vi "DPID.CheckErrors.vi"(6 "Existing PIDs":T1[](array[typedef]) {"Signals"."Byte Order" items=["Little Endian", "Big Endian"]; "Signals"."Data Type" items=["Signed", "Unsigned", "IEEE Float"]}, 8 "error in (no error)":errorcluster, 9 "Existing DPIDs":u8[](array[numeric]), 10 "DPID ID":u8, 11 "PIDs":u16[](array[numeric])) -> (0 "error out":errorcluster, 2 "Reason":string, 3 "Error?":bool)   [LabVIEW 2019, in "Diagnostics Addon System Explorer.lvlib"]
uses:
  Diagnostics Addon System Explorer.lvlib
  Types/Frame.Export.ctl
  Shared/Types/Signal.ctl
  Shared/Diagnostics Addon Shared.lvlib
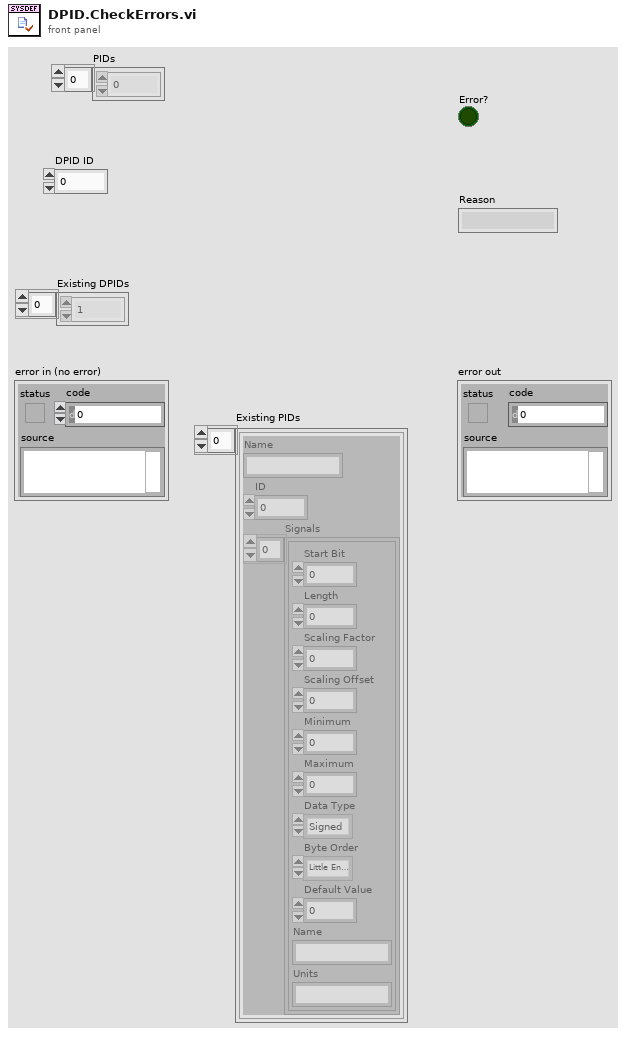
[diagram p1: front panel]
types:
  T1 = typedef "Diagnostics Addon System Explorer.lvlib/Frame.Export.ctl" = cluster{"Name":string, "ID":u32, "Signals":T2[]}
  T2 = typedef "Diagnostics Addon Shared.lvlib/Signal.ctl" = cluster{"Start Bit":u32, "Length":u32, "Scaling Factor":dbl, "Scaling Offset":dbl, "Minimum":dbl, "Maximum":dbl, "Data Type":u32, "Byte Order":u32, "Default Value":dbl, "Name":string, "Units":string}
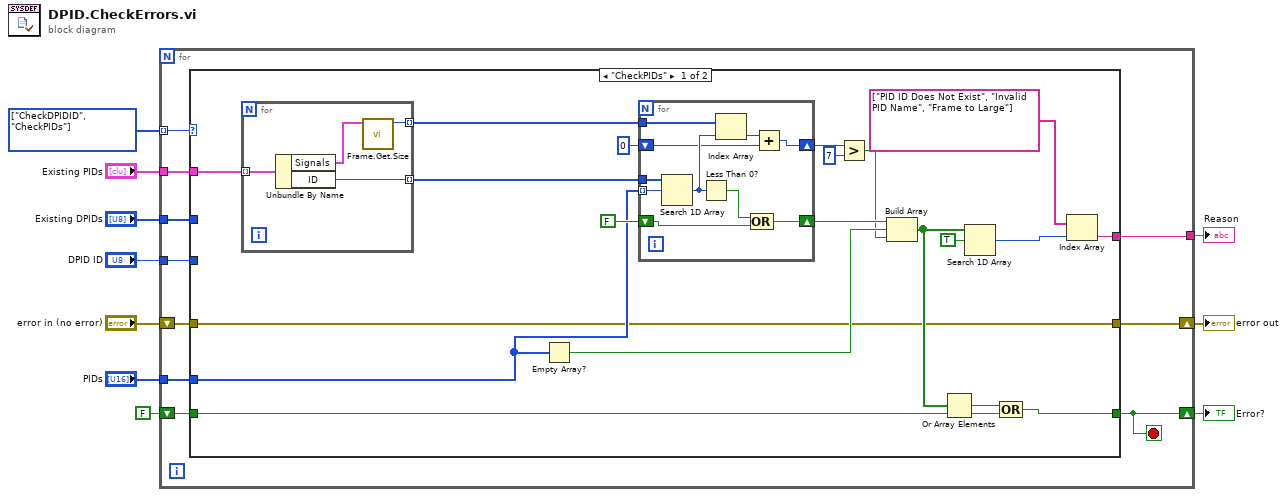
[diagram p0: block diagram]
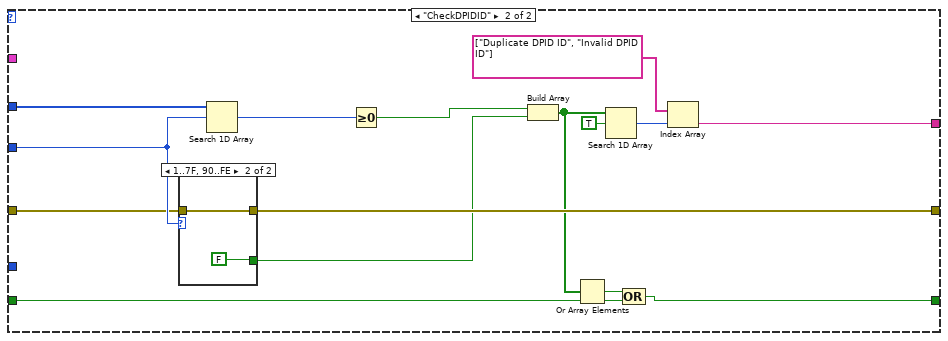
[diagram p2: hidden frame]
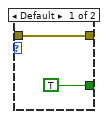
[diagram p3: hidden frame]
diagram:
  w10 = enum16{"CheckDPIDID", "CheckPIDs"}[] [enum."CheckDPIDID", enum."CheckPIDs"] items=["CheckDPIDID", "CheckPIDs"]
  n1 = for {
    tunnel: w10 -> [w20] mode=indexing
    shift-right: [w18] -> w8
    shift-left: "error in (no error)" -> [w19]
    tunnel: "Existing DPIDs" -> [w17]
    shift-right: [w14] -> w5
    shift-left: FALSE -> [w16]
    tunnel: [w15] -> w4
    tunnel: "Existing PIDs" -> [w13]
    tunnel: "PIDs" -> [w12]
    tunnel: "DPID ID" -> [w11]
    stop <- w14 stop-if-true
    n2 = case shown="\"CheckPIDs\"" w20 {
      tunnel: w19 -> [w21 w55]
      tunnel: [w21 w69] -> w18
      tunnel: w17 -> [_ w68]
      tunnel: [w38 w65] -> w14
      tunnel: w16 -> [w39 w66]
      tunnel: [w32 w57] -> w15
      tunnel: w13 -> [w28 _]
      tunnel: w12 -> [w22 _]
      tunnel: w11 -> [_ w56]
      frame "CheckPIDs" {
        n3 = for {
          tunnel: [w41] -> w40 mode=indexing
          tunnel: w28 -> [w44] mode=indexing
          tunnel: [w43] -> w27 mode=indexing
          n4 = Unbundle By Name(w44) -> ("Signals"=w42:T2[], "ID"=w41:u32)
          n5 = call "Frame.Get.Size.vi"("Parameters"=w42) -> ("Bytes"=w43:u32)  [unwired: 10 in]
        }
        n6 = Empty Array?(array=w22) -> (empty?=w30:bool)
        n7 = for {
          tunnel: w40 -> [w54]
          tunnel: w22 -> [w53] mode=indexing
          shift-right: [w51] -> w34
          shift-left: FALSE -> [w50]
          tunnel: w27 -> [w49]
          shift-right: [w46] -> w25
          shift-left: u8 0 ("Frame Length") -> [w45]
          n8 = Search 1D Array(1D array=w54, element=w53) -> (index of element=w48:i32)  [unwired: 1 in]
          n9 = Less Than 0?(x=w48) -> (x < 0?=w52:bool)
          n10 = Index Array(array=w49, index=w48) -> (element=w47:u32)
          n11 = Compound Arithmetic op=OR(w52, w50) -> (w51:bool)
          n12 = Add(x=w47, y=w45) -> (x+y=w46:u32)
        }
        n13 = Greater?(x=w25, y=u8 7) -> (0:w23:bool)
        n14 = Build Array(w34, w30, w23) -> (w31:bool[])
        n15 = Or Array Elements(Boolean array=w31) -> (logical OR=w29:bool)
        n16 = Search 1D Array(1D array=w31, element=TRUE) -> (index of element=w36:i32)  [unwired: 1 in]
        n17 = Compound Arithmetic op=OR(w29, w39) -> (w38:bool)
        n18 = Index Array(array=string[] ["PID ID Does Not Exist", "Invalid PID Name", "Frame to Large"], index=w36) -> (element=w32:string)
      }
      frame "CheckDPIDID" {
        n19 = case shown="1..7F, 90..FE" w56 {
          tunnel: [w71 w73] -> w69
          tunnel: w55 -> [w71 w73]
          tunnel: [TRUE FALSE] -> w59
          frame Default {
          }
          frame 1..127, 144..254 {
          }
        }
        n20 = Search 1D Array(1D array=w68, element=w56) -> (index of element=w67:i32)  [unwired: 1 in]
        n21 = Greater Or Equal To 0?(x=w67) -> (x >= 0?=w60:bool)
        n22 = Build Array(w60, w59) -> (w61:bool[])
        n23 = Or Array Elements(Boolean array=w61) -> (logical OR=w58:bool)
        n24 = Search 1D Array(1D array=w61, element=TRUE) -> (index of element=w63:i32)  [unwired: 1 in]
        n25 = Compound Arithmetic op=OR(w58, w66) -> (w65:bool)
        n26 = Index Array(array=string[] ["Duplicate DPID ID", "Invalid DPID ID"], index=w63) -> (element=w57:string)
      }
    }
  }
  "error out" <- w8
  "Error?" <- w5
  "Reason" <- w4
